vi "dfd_Merge FLP and FXP Analysis Outputs.vi"(4 "delta":dbl, 7 "output option":u16(ring) items=["Auto", "Floating-Point Only", "Fixed-Point Only"], 8 "error in FXP":errorcluster, 9 "response FXP":dbl[](array[numeric]) format="%.2f", 10 "error in FLP":errorcluster, 11 "response FLP":dbl[](array[numeric]) format="%.2f") -> (0 "error out":errorcluster, 2 "time responses":T1(array[cluster]) {"dt" format="%.2f"; "t0" format="%.2f"; "amplitudes" format="%.2f"}, 3 "freq responses":cluster{"f0":dbl, "df":dbl, "values":dbl[]}[](array[cluster]) {"df" format="%.2f"; "f0" format="%.2f"; "values" format="%.2f"})   [LabVIEW 2017, in "NI_DigFilterLicensed.lvlib"]
uses:
  <vilib>/addons/Digital Filter Design/NI_DigFilterLicensed.lvlib
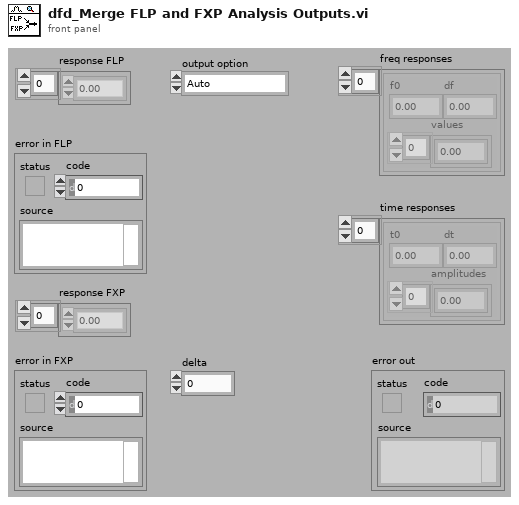
[diagram p1: front panel]
types:
  T1 = cluster{"t0":dbl, "dt":dbl, "amplitudes":dbl[]}[]
  T2 = cluster{dbl, "delta":dbl, "response FXP":dbl[]}[]
  T3 = cluster{dbl, "delta":dbl, "response FLP":dbl[]}[]
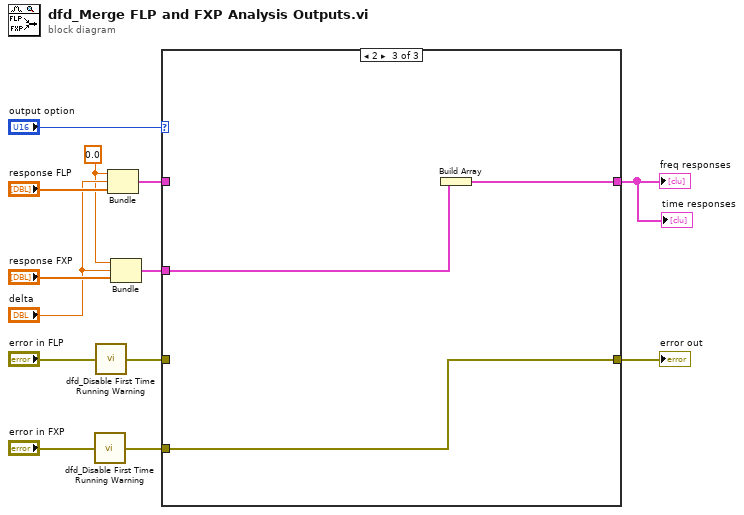
[diagram p0: block diagram]
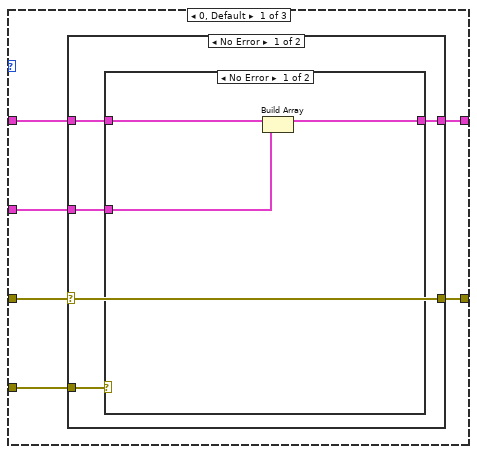
[diagram p2: hidden frame]
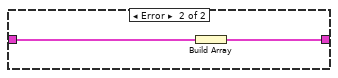
[diagram p3: hidden frame]
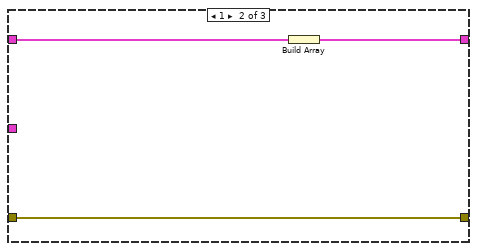
[diagram p5: hidden frame]
diagram:
  w5 = 0.0
  n1 = call <vilib>:"dfd_Disable First Time Running Warning.vi"("error in"="error in FXP") -> ("error out"=w2:errorcluster)  [unwired: 1 in]
  n2 = call <vilib>:"dfd_Disable First Time Running Warning.vi"("error in"="error in FLP") -> ("error out"=w4:errorcluster)  [unwired: 1 in]
  n3 = Bundle(w5, "delta"="delta", "response FLP"="response FLP") -> (w9:cluster{dbl, "delta":dbl, "response FLP":dbl[]})  [unwired: 1 out]
  n4 = Bundle(w5, "delta"="delta", "response FXP"="response FXP") -> (w6:cluster{dbl, "delta":dbl, "response FXP":dbl[]})  [unwired: 1 out]
  n5 = case shown="2" "output option" {
    tunnel: w9 -> [w17 w33 _]
    tunnel: w6 -> [w15 _ w35]
    tunnel: w4 -> [w19 w31 _]
    tunnel: w2 -> [w18 _ w34]
    tunnel: [w16 w32 w36] -> w1
    tunnel: [w14 w31 w34] -> w11
    frame 0, Default {
      n6 = case shown="No Error" w19 {
        selector: w19 -> [w20 w30]
        tunnel: w18 -> [w24 _]
        tunnel: w17 -> [w23 _]
        tunnel: [w22 _] -> w16
        tunnel: w15 -> [w21 _]
        tunnel: [w20 w30] -> w14
        frame No Error {
          n7 = case shown="No Error" w24 {
            tunnel: w23 -> [w27 w29]
            tunnel: [w25 w28] -> w22
            tunnel: w21 -> [w26 _]
            frame No Error {
              n8 = Build Array(w27, w26) -> (w25:T2)
            }
            frame Error {
              n9 = Build Array(w29) -> (w28:T3)
            }
          }
        }
        frame Error {
        }
      }
    }
    frame 1 {
      n10 = Build Array(w33) -> (w32:T3)
    }
    frame 2 {
      n11 = Build Array(w35) -> (w36:T2)
    }
  }
  "error out" <- w11
  "freq responses" <- w1
  "time responses" <- w1
